vi "List Components.vi"(8 "error in (no error)":errorcluster, 11 "reserved":string) -> (0 "error out":errorcluster, 2 "Components":string[](array[string]), 3 "reserved dup":string)   [LabVIEW 2021, in "smo.lvlib" / "SMOFacade.lvclass"]
uses:
  SMOFacade.lvclass
  SMOFacade.lvclass/SMOFacade.ctl
  Registry/Registry-SMO.lvclass
  SMO/SMO.lvclass
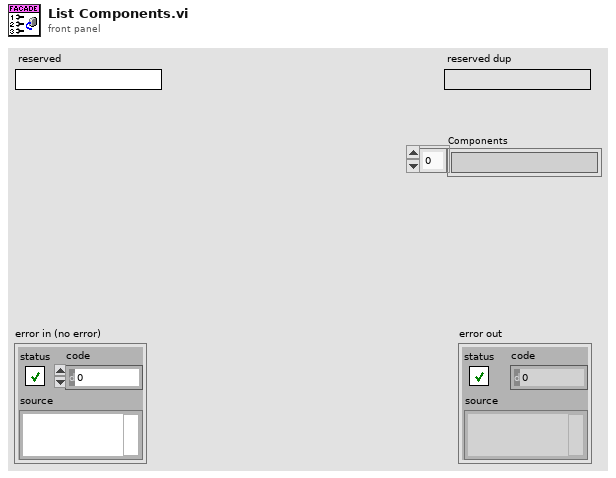
[diagram p1: front panel]
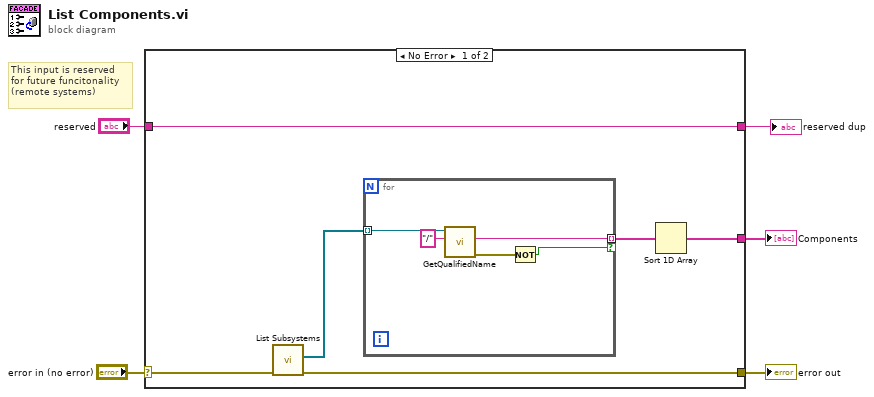
[diagram p0: block diagram]
diagram:
  # "This input is reserved\nfor future funcitonality\n(remote systems)"
  n1 = case shown="No Error" "error in (no error)" {
    selector: "error in (no error)" -> [w11 w18]
    tunnel: [w10 w18] -> w4
    tunnel: "reserved" -> [w6 w17]
    tunnel: [w7 _] -> w2
    tunnel: [w6 w17] -> w1
    frame No Error {
      n2 = call "List Subsystems.vi"("error in (no error)"=w11) -> ("error out"=w10:errorcluster, "Subsystems"=w9:refnum<class "SMO.lvclass">[])  [unwired: 9 in]
      n3 = for {
        tunnel: w9 -> [w16] mode=indexing
        tunnel: [w14] -> w8 mode=indexing if=w12
        n4 = call "GetQualifiedName.vi"("separator (dot)"="/", "SMO"=w16) -> ("error out"=w13:errorcluster, "Qualified Name"=w14:string)  [unwired: 7 in, 1 out]
        n5 = Not(x=w13) -> (.not. x?=w12:bool)
      }
      n6 = Sort 1D Array(array=w8) -> (sorted array=w7:string[])
    }
    frame Error {
    }
  }
  "error out" <- w4
  "Components" <- w2
  "reserved dup" <- w1
